vi "read-text.vi"() -> ()   [LabVIEW 2020]
uses:
  <vilib>/userDefined/High Color/IMAQdx.ctl
  <vilib>/vision/driver/NI_Vision_Acquisition_Software.lvlib
  <vilib>/vision/NI_Vision_Development_Module.lvlib
panel:
  out "Read String":string
  in  "Rectangle":T1 {"Rotation" min=-90.0 max=90.0 step=1.0 format="%.2f"; "Left" scale=0.0..1024.0; "Right" scale=0.0..1024.0}
  out "Image":T2(plugin-control)
  in  "Session In":T3
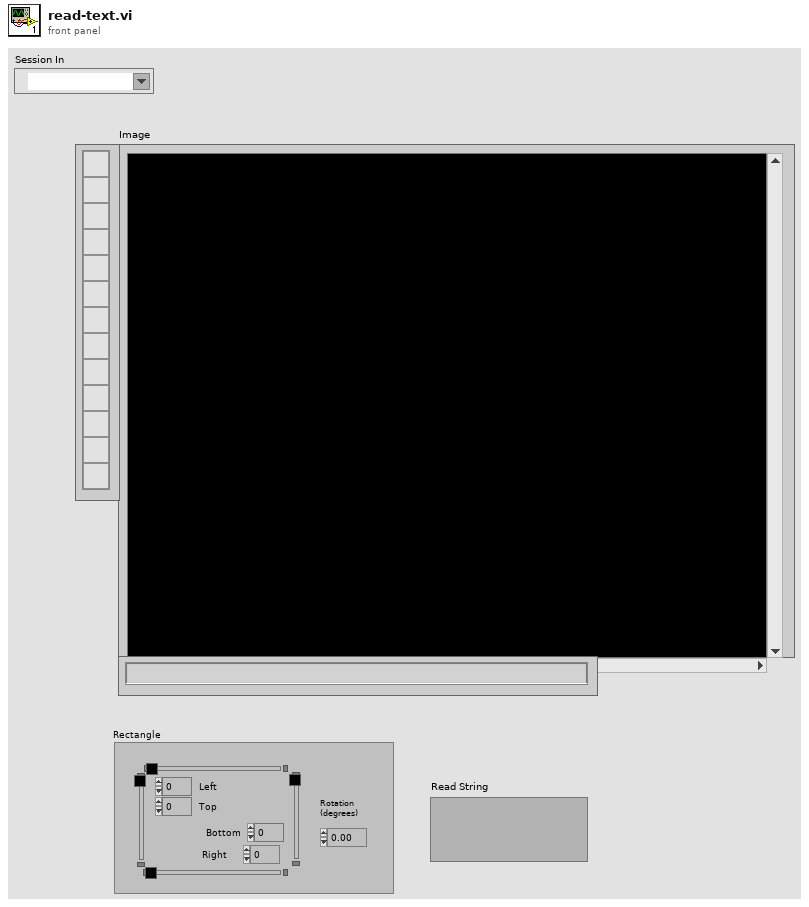
[diagram p1: front panel]
types:
  T1 = typedef "IMAQ Rectangle" = cluster{"Left":i32, "Top":i32, "Right":i32, "Bottom":i32, "Rotation":dbl}
  T2 = typedef "IMAQ Image.ctl" = refnum<image>
  T3 = typedef "IMAQdx.ctl" = refnum<k21>
  T4 = typedef "IMAQ OCR Session.ctl" = refnum<k1>
  T5 = typedef "ROI Descriptor" = cluster{"Global Rectangle":i32[], "Contours":cluster{"ID":enum32{"External", "Internal"}, "Type":u32, "Coordinates":i32[]}[]}
  T6 = cluster{"Global Rectangle":i32[], "Contours":cluster{"ID":enum32{"External", "Internal"}, "Type":u32, "Coordinates":i32[]}[]}
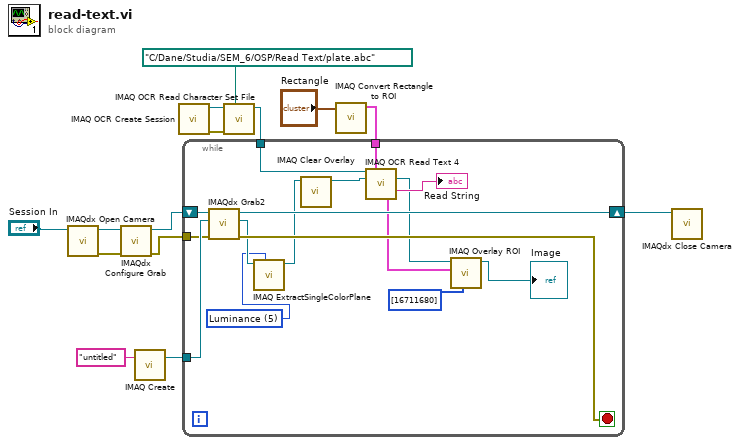
[diagram p0: block diagram]
diagram:
  n1 = call <vilib>:"IMAQdx Open Camera.vi"("Session In"="Session In") -> ("error out"=w13:errorcluster, "Session Out"=w14:T3)  [unwired: 9 in]
  n2 = call <vilib>:"IMAQdx Configure Grab.vi"("error in"=w13, "Session In"=w14) -> ("error out"=w9:errorcluster, "Session Out"=w12:T3)  [unwired: 8 in]
  n3 = call "IMAQ Create"("Image Name"="untitled") -> ("New Image"=w10:T2)  [unwired: 4 in, 1 out]
  n4 = call "IMAQ OCR Create Session"() -> ("error out"=w6:errorcluster, "IMAQ OCR Session"=w5:T4)  [unwired: 10 in]
  n5 = call "IMAQ OCR Read Character Set File"("File Path"=path "C:/Dane/Studia/SEM_6/OSP/Read Text/plate.abc", "error in (no error)"=w6, "IMAQ OCR Session"=w5) -> ("IMAQ OCR Session (dup)"=w3:T4)  [unwired: 6 in, 2 out]
  n6 = call "IMAQ Convert Rectangle to ROI"("Rectangle"="Rectangle") -> ("ROI Descriptor"=w1:T5)  [unwired: 8 in, 1 out]
  n7 = while {
    tunnel: w10 -> [w29]
    tunnel: w9 -> [w28]
    shift-right: [w27] -> w8
    shift-left: w12 -> [w30]
    tunnel: w3 -> [w26]
    tunnel: w1 -> [w25]
    stop <- w23 stop-if-true
    w15 = 5 items=["Red", "Green", "Blue", "Hue", "Saturation", "Luminance", "Value", "Intensity"] ("Color Plane")
    n8 = call <vilib>:"IMAQdx Grab2.vi"("error in"=w28, "Image In"=w29, "Session In"=w30) -> ("error out"=w23:errorcluster, "Image Out"=w17:T2, "Session Out"=w27:T3)  [unwired: 5 in, 1 out]
    n9 = call "IMAQ ExtractSingleColorPlane"("Color Plane"=w15, "Image Src"=w17) -> ("Image Dst Out"=w16:T2)  [unwired: 2 in, 7 out]
    n10 = call "IMAQ Clear Overlay"("Image"=w16) -> ("Image Out"=w18:T2)  [unwired: 9 in, 1 out]
    n11 = call "IMAQ OCR Read Text 4"("IMAQ OCR Session"=w26, "ROI Descriptor"=w25, "Image"=w18) -> ("Image (dup)"=w21:T2, "Read String"=→"Read String":string, "ROI Bounding Characters"=w20:T6)  [unwired: 6 in, 4 out]
    n12 = call "IMAQ Overlay ROI"("Colors (Green)"=u32[] [16711680], "ROI Descriptor"=w20, "Image"=w21) -> ("Image Out"=→"Image":T2)  [unwired: 7 in, 1 out]
  }
  n13 = call <vilib>:"IMAQdx Close Camera.vi"("Session In"=w8) -> ()  [unwired: 10 in, 1 out]
